vi "Auto Gear Align 2.0.vi"(8 "Error In":errorcluster, 10 "Camera Image":T2, 11 "Refnum's In":T1={"RobotDrive"="RobotDrive", "Gyro"="Gyro", "Mtr 1"="LeftMtr", "Mtr 2"="RightMtr"}) -> (0 "Error Out":errorcluster, 3 "Refnum's Out":T1={"RobotDrive"="RobotDrive", "Gyro"="Gyro", "Mtr 1"="LeftMtr", "Mtr 2"="RightMtr"})   [LabVIEW 2016]
uses:
  <vilib>/vision/Image Controls.llb/IMAQ Image.ctl
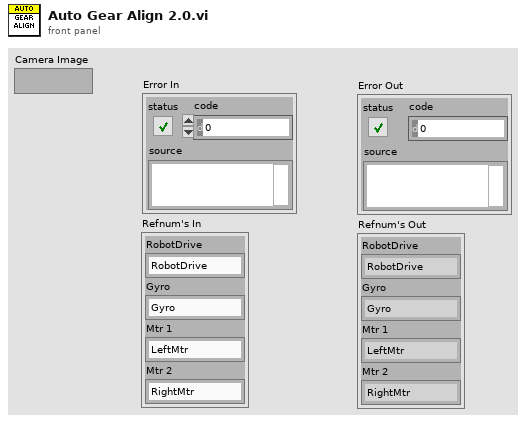
[diagram p1: front panel]
types:
  T1 = cluster{"RobotDrive":string, "Gyro":string, "Mtr 1":string, "Mtr 2":string}
  T2 = typedef "IMAQ Image.ctl" = refnum<image>
  T3 = typedef "WPI_JoystickDevRef.ctl" = cluster{"Device":T4}
  T4 = typedef "WPI_JoystickDeviceEnum.ctl" = enum16{"USB 0", "USB 1", "USB 2", "USB 3", "USB 4", "USB 5"}
  T5 = cluster{"Left":dbl, "Top":dbl, "Right":dbl, "Bottom":dbl}
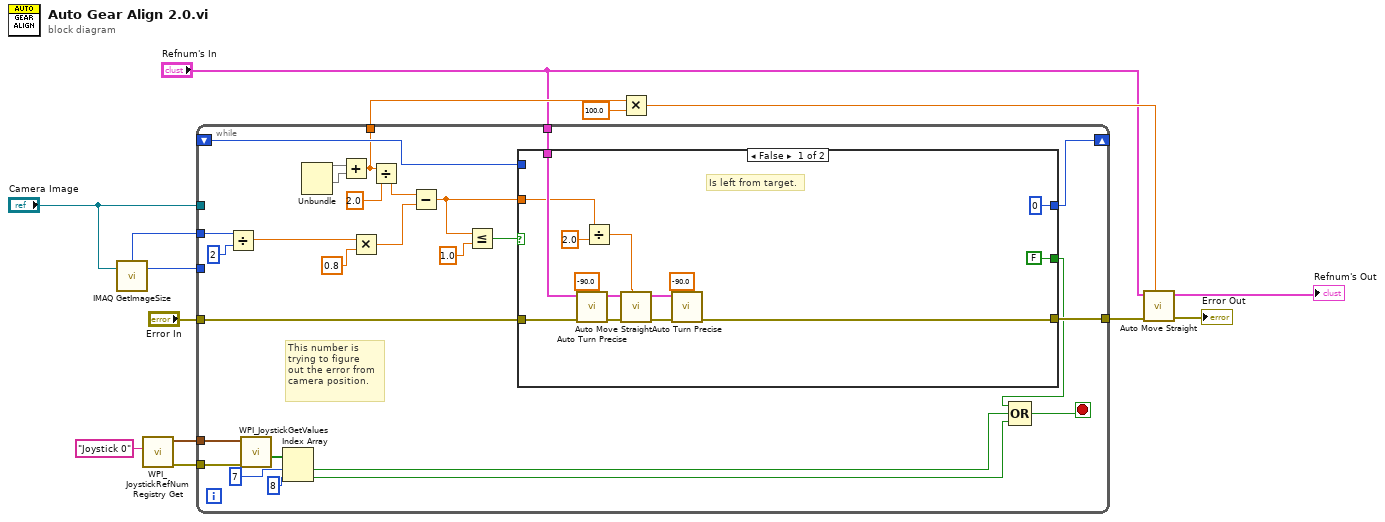
[diagram p0: block diagram]
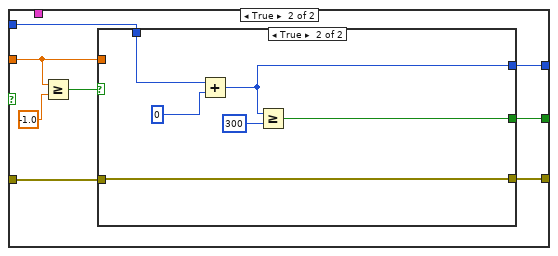
[diagram p2: hidden frame]
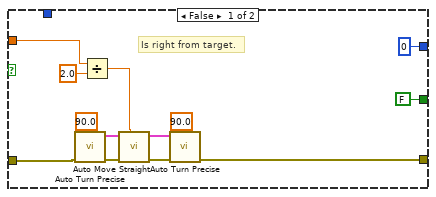
[diagram p3: hidden frame]
diagram:
  n1 = call "IMAQ GetImageSize"("Image"="Camera Image") -> ("Y Resolution"=w13:i32, "X Resolution"=w12:i32)  [unwired: 3 in, 1 out]
  n2 = call <vilib>:"WPI_JoystickRefNum Registry Get.vi"("refnum name"="Joystick 0") -> ("error out"=w1:errorcluster, "JoystickDevRef"=w2:T3)  [unwired: 9 in]
  n3 = while {
    tunnel: "Camera Image" -> [w43]
    tunnel: w13 -> [_]
    tunnel: w12 -> [w41]
    tunnel: "Refnum's In" -> [w34]
    shift-right: [w28] -> _
    shift-left: _ -> [w27]
    tunnel: [w26] -> w11
    tunnel: "Error In" -> [w25]
    tunnel: [w24] -> w6
    tunnel: w2 -> [w20]
    tunnel: w1 -> [w19]
    stop <- w17 stop-if-true
    # "This number is \ntrying to figure\nout the error from\ncamera position."
    n4 = Divide(x=w41, y=2) -> (x/y=w39:dbl)
    n5 = call <vilib>:"WPI_JoystickGetValues.vi"("error in (no error)"=w19, "JoystickDevRef"=w20) -> ("Buttons"=w23:bool[])  [unwired: 5 in, 4 out]
    n6 = Index Array(array=w23, index #1=7 ("index"), index #2=8 ("index")) -> (element #1=w16:bool, element #2=w15:bool)
    n7 = Unbundle() -> (w42:T5, "Left"=w37, "Right"=w36)  [unwired: 2 out]
    n8 = Add(x=w37, y=w36) -> (x+y=w26:dbl)
    n9 = Multiply(x=w39, y=0.8) -> (x*y=w32:dbl)
    n10 = Divide(x=w26, y=2.0) -> (x/y=w33:dbl)
    n11 = Subtract(x=w33, y=w32) -> (x-y=w30:dbl)
    n12 = Less Or Equal?(x=w30, y=1.0) -> (x <= y?=w31:bool)
    n13 = case shown="False" w31 {
      tunnel: w34 -> [w57 _]
      tunnel: w30 -> [w53 w63]
      tunnel: [0 w62] -> w28
      tunnel: w27 -> [_ w61]
      tunnel: [FALSE w60] -> w18
      tunnel: w25 -> [w45 w59]
      tunnel: [w44 w58] -> w24
      frame False {
        # "Is left from target."
        n14 = call "Auto Turn Precise.vi"("Target Distance"=-90.0, "Error In"=w45, "Refnum's In"=w57) -> ("Error Out"=w55:errorcluster, "Refnum's Out"=w54:T1)  [unwired: 7 in]
        n15 = Divide(x=w53, y=2.0) -> (x/y=w51:dbl)
        n16 = call "Auto Move Straight.vi"("Target Distance"=w51, "Error In"=w55, "Refnum's In"=w54) -> ("Error Out"=w49:errorcluster, "Refnum's Out"=w48:T1)  [unwired: 7 in]
        n17 = call "Auto Turn Precise.vi"("Target Distance"=-90.0, "Error In"=w49, "Refnum's In"=w48) -> ("Error Out"=w44:errorcluster)  [unwired: 7 in, 1 out]
      }
      frame True {
        n18 = Greater Or Equal?(x=w63, y=-1.0) -> (x >= y?=w64:bool)
        n19 = case shown="True" w64 {
          tunnel: w63 -> [w70 _]
          tunnel: w61 -> [_ w84]
          tunnel: [0 w81] -> w62
          tunnel: [FALSE w80] -> w60
          tunnel: w59 -> [w67 w79]
          tunnel: [w66 w79] -> w58
          frame False {
            # "Is right from target."
            n20 = call "Auto Turn Precise.vi"("Target Distance"=90.0, "Error In"=w67) -> ("Error Out"=w77:errorcluster, "Refnum's Out"=w76:T1)  [unwired: 8 in]
            n21 = Divide(x=w70, y=2.0) -> (x/y=w74:dbl)
            n22 = call "Auto Move Straight.vi"("Target Distance"=w74, "Error In"=w77, "Refnum's In"=w76) -> ("Error Out"=w72:errorcluster, "Refnum's Out"=w71:T1)  [unwired: 7 in]
            n23 = call "Auto Turn Precise.vi"("Target Distance"=90.0, "Error In"=w72, "Refnum's In"=w71) -> ("Error Out"=w66:errorcluster)  [unwired: 7 in, 1 out]
          }
          frame True {
            n24 = Add(x=w84, y=0) -> (x+y=w81:i32)
            n25 = Greater Or Equal?(x=w81, y=300) -> (x >= y?=w80:bool)
          }
        }
      }
    }
    n26 = Compound Arithmetic op=OR(w18, w16, w15) -> (w17:bool)
  }
  n27 = Multiply(x=w11, y=100.0) -> (x*y=w9:dbl)
  n28 = call "Auto Move Straight.vi"("Target Distance"=w9, "Error In"=w6, "Refnum's In"="Refnum's In") -> ("Error Out"=→"Error Out":errorcluster, "Refnum's Out"=→"Refnum's Out":T1)  [unwired: 7 in]
